vi "uStringManipulation_DO.vi"(8 "error in (no error)":errorcluster, 10 "String in":string, 11 "in":refnum<class "replacePrefix.lvclass">) -> (0 "error out":errorcluster, 2 "String":string, 3 "out":refnum<class "replacePrefix.lvclass">)   [LabVIEW 2023, in "uStringManipulation_Pack_Std.lvlib" / "replacePrefix.lvclass"]
uses:
  replacePrefix.lvclass
  replacePrefix.lvclass/replacePrefix.ctl
  <vilib>/ErrorRing/Error Ring.xnode
  <vilib>/Utility/error.llb/Error Cluster From Error Code.vi
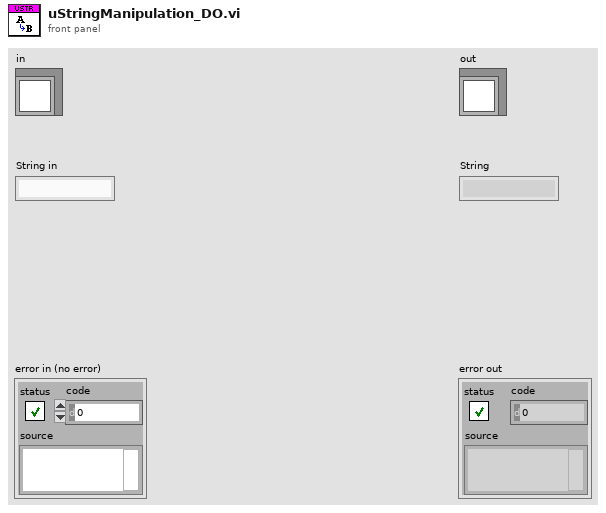
[diagram p1: front panel]
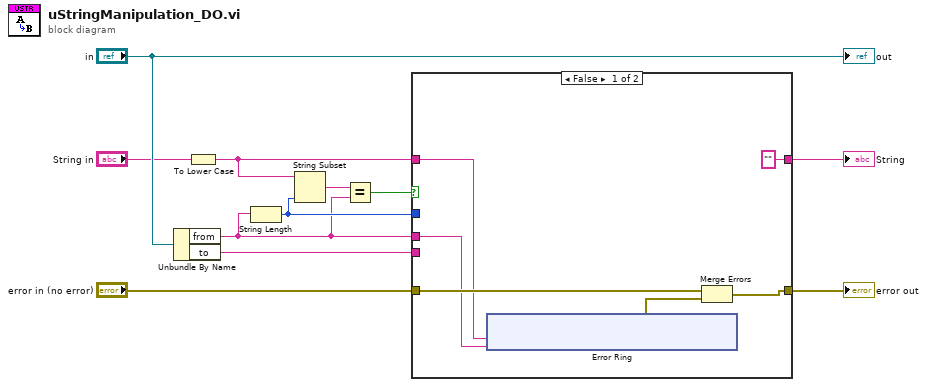
[diagram p0: block diagram]
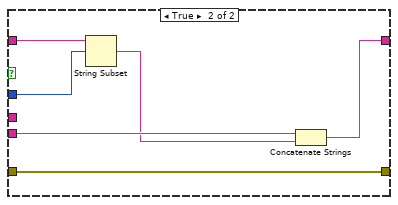
[diagram p2: hidden frame]
diagram:
  n1 = Unbundle By Name("in") -> ("from"=w1:string, "to"=w3:string)
  n2 = To Lower Case(string="String in") -> (all lower case string=w7:string)
  n3 = String Length(string=w1) -> (length=w2:i32)
  n4 = String Subset(string=w7, length (rest)=w2) -> (substring=w6:string)  [unwired: 1 in]
  n5 = Equal?(x=w6, y=w1) -> (x = y?=w5:bool)
  n6 = case shown="False" w5 {
    tunnel: w7 -> [w13 w29]
    tunnel: ["" w30] -> w11
    tunnel: [w15 w31] -> w10
    tunnel: "error in (no error)" -> [w16 w31]
    tunnel: w3 -> [_ w28]
    tunnel: w2 -> [_ w26]
    tunnel: w1 -> [w12 _]
    frame False {
      n7 = xnode "Error Ring"("parameter 0"=w13, "parameter 1"=w12) -> ("error out"=w14:errorcluster)
      n8 = Merge Errors(w16, w14) -> (w15:errorcluster)
    }
    frame True {
      n9 = String Subset(string=w29, offset (0)=w26) -> (substring=w27:string)  [unwired: 1 in]
      n10 = Concatenate Strings(w28, w27) -> (w30:string)
    }
  }
  "error out" <- w10
  "String" <- w11
  "out" <- "in"
